vi "Requests.vi"(8 "error in (no error)":errorcluster, 9 "write enable":bool=TRUE, 11 "ICPCON ET-7028 in":refnum<class "ICPCON ET-7028.lvclass">) -> (0 "error out":errorcluster, 3 "ICPCON ET-7028 out":refnum<class "ICPCON ET-7028.lvclass">)   [LabVIEW 2021, in "ICPCON ET-7028.lvclass"]
uses:
  ICPCON ET-7028.lvclass
  D:/my_projects/projects/Algorithms/Labview/21/Modbus/MB_TCP2/MB_TCP.lvclass
  MB_TCP.lvclass/MB_TCP.ctl
  NI_modbus_upd/Ctl/Unit_ID.ctl
  NI_modbus_upd/TCP/TCP.lvclass/TCP.ctl
  NI_modbus_upd/Master Function Definition/Responses/Read Holding Registers Response.vi
  NI_modbus_upd/Master Function Definition/Requests/Read Holding Registers Request.vi
  NI_modbus_upd/Master network read write.vi
  NI_modbus_upd/Function data mismatch error1.vi
  NI_modbus_upd/Master Function Definition/Responses/Write Multiple Registers Response.vi
  NI_modbus_upd/Master Function Definition/Requests/Write Multiple Registers Request.vi
  NI_modbus_upd/Utility/Bytes to U16s1.vi
  NI_modbus_upd/Function code mismatch error1.vi
  NI_modbus_upd/Error Generator1.vi
  NI_modbus_upd/Modbus Data Unit (PDU)/Construct PDU1.vi
  NI_modbus_upd/Read ADU Packet Master.vi
  NI_modbus_upd/Write ADU Packet Master.vi
  NI_modbus_upd/Utility/U16s to Bytes1.vi
  NI_modbus_upd/Modbus Data Unit (PDU)/Unflatten to PDU1.vi
  NI_modbus_upd/TCP/Protocol Read.vi
  NI_modbus_upd/TCP/Protocol Write.vi
  <vilib>/Utility/error.llb/Clear Errors.vi
  NI_modbus_upd/Modbus Data Unit (PDU)/Deconstruct PDU1.vi
  NI_modbus_upd/TCP/TCP.lvclass
  ICPCON Registers/ICPCON Registers.lvlib
  MB_TCP.lvclass
  NI_modbus_upd/NI_modbus_upd.lvlib
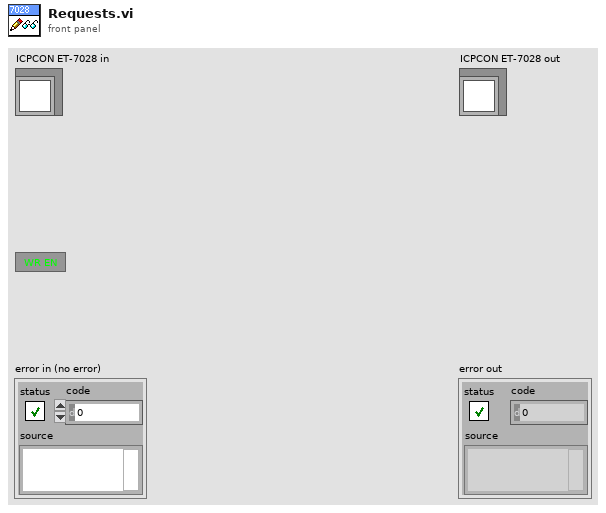
[diagram p1: front panel]
types:
  T1 = typedef "NI_modbus_upd.lvlib/Unit_ID.ctl" = cluster{"Protocol ID":u16, "Unit ID":u8}
  T2 = typedef "ICPCON Registers.lvlib/ICPCON Data.ctl" = cluster{"UTF":refnum<data-value>, "DI":refnum<data-value>, "DW":refnum<data-value>, "DO":refnum<data-value>, "IR":refnum<data-value>, "WR":refnum<data-value>, "OR":refnum<data-value>, "modified":refnum<data-value>}
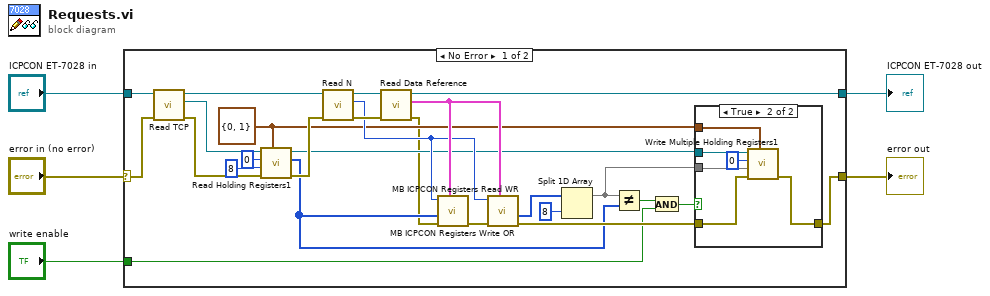
[diagram p0: block diagram]
diagram:
  n1 = case shown="No Error" "error in (no error)" {
    selector: "error in (no error)" -> [w25 w40]
    tunnel: [w16 w40] -> w3
    tunnel: [w23 w39] -> w4
    tunnel: "ICPCON ET-7028 in" -> [w26 w39]
    tunnel: "write enable" -> [w12 _]
    frame No Error {
      w8 = T1 {"Protocol ID"=0, "Unit ID"=1} ("Unit_ID")
      n2 = call "Read TCP.vi"("error in (no error)"=w25, "MB_TCP in"=w26) -> ("error out"=w9:errorcluster, "TCP"=w10:refnum<class "TCP.lvclass">, "MB_TCP out"=w27:refnum<class "ICPCON ET-7028.lvclass">)  [unwired: 7 in]
      n3 = call "Read Holding Registers1.vi"("Unit_ID"=w8, "error in (no error)"=w9, "number of holding registers"=u16 8 ("number of discrete inputs"), "starting address"=u16 0, "Modbus master in"=w10) -> ("error out"=w24:errorcluster, "register values"=w11:u16[], "Modbus master out"=w7:refnum<class "TCP.lvclass">)  [unwired: 4 in]
      n4 = call "Read N.vi"("error in (no error)"=w24, "MB_TCP in"=w27) -> ("error out"=w30:errorcluster, "N"=w13:i32, "MB_TCP out"=w31:refnum<class "ICPCON ET-7028.lvclass">)  [unwired: 7 in]
      n5 = call "Read Data Reference.vi"("error in (no error)"=w30, "MB_TCP in"=w31) -> ("error out"=w6:errorcluster, "Data"=w14:T2, "MB_TCP out"=w23:refnum<class "ICPCON ET-7028.lvclass">)  [unwired: 7 in]
      n6 = call "MB ICPCON Registers Write OR.vi"("Data Reference"=w14, "error in (no error)"=w6, "Words In"=w11, "N"=w13) -> ("error out"=w15:errorcluster)  [unwired: 7 in]
      n7 = call "MB ICPCON Registers Read WR.vi"("Data Reference"=w14, "error in (no error)"=w15, "N"=w13) -> ("error out"=w17:errorcluster, "Words out"=w21:u16[])  [unwired: 7 in]
      n8 = Split 1D Array(array=w21, index=8 ("length")) -> (first subarray=w18:u16[])  [unwired: 1 out]
      n9 = Not Equal?(x=w18, y=w11) -> (x != y?=w20:bool)
      n10 = And(x=w20, y=w12) -> (x .and. y?=w19:bool)
      n11 = case shown="True" w19 {
        tunnel: w17 -> [w32 w37]
        tunnel: [w32 w35] -> w16
        tunnel: w7 -> [_ w38]
        tunnel: w8 -> [_ w33]
        tunnel: w18 -> [_ w34]
        frame False {
        }
        frame True {
          n12 = call "Write Multiple Holding Registers1.vi"("Unit_ID"=w33, "error in (no error)"=w37, "holding register values"=w34, "starting address"=u16 0, "Modbus master in"=w38) -> ("error out"=w35:errorcluster)  [unwired: 5 in, 1 out]
        }
      }
    }
    frame Error {
    }
  }
  "error out" <- w3
  "ICPCON ET-7028 out" <- w4
